vi "OriginSearch.vi"(8 "error in":errorcluster, 11 "VISA resource":refnum<visa-resource-name>) -> (0 "error out":errorcluster)   [LabVIEW 2012, in "Micos_uic.lvlib"]
uses:
  <instrlib>/Micos_uic/Micos_uic.lvlib
  <vilib>/Utility/error.llb/DialogType.ctl
panel:
  out "Itration":i32
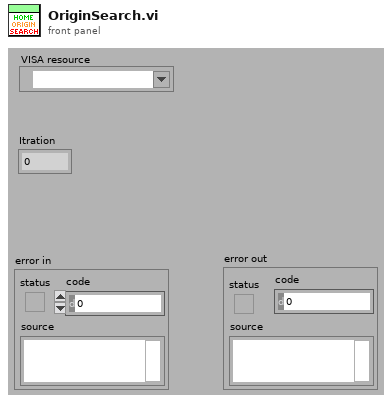
[diagram p1: front panel]
types:
  T1 = typedef "DialogType.ctl" = u16
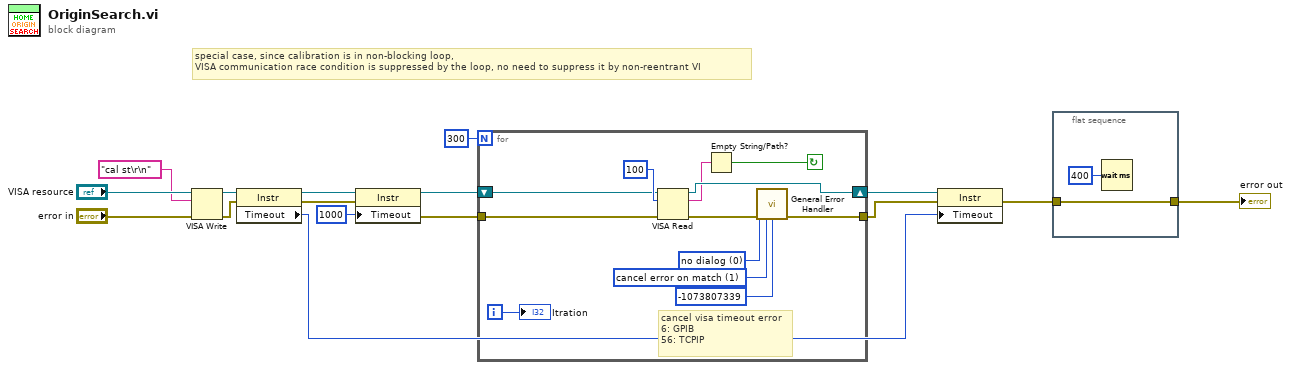
[diagram p0: block diagram]
diagram:
  # "special case, since calibration is in non-blocking loop,\nVISA communication race condition is suppressed by the loop, no need to suppress it by non-reentrant VI"
  n1 = VISA Write(VISA resource name="VISA resource", write buffer="cal st\r\n", error in (no error)="error in") -> (VISA resource name out=w13:refnum<visa-resource-name>, error out=w10:errorcluster)  [unwired: 1 out]
  n2 = property class="Instr"(reference=w13, error in=w10) -> (reference out=w12:refnum<visa-resource-name>, error out=w9:errorcluster, "Timeout"=w6:u32)
  n3 = property class="Instr"(reference=w12, error in=w9, "Timeout"=u32 1000 ("General Settings:Timeout Value")) -> (reference out=w11:refnum<visa-resource-name>, error out=w8:errorcluster)
  n4 = for {
    N: 300 -> [_]
    tunnel: w8 -> [w20]
    tunnel: [w25] -> w4
    shift-right: [w26] -> w7
    shift-left: w11 -> [w19]
    i -> [w18]
    stop <- w21 continue-if-true
    w17 = T1 0 items=["no dialog", "OK message", "continue or stop message", "OK message + warnings", "continue/stop + warnings"] ("type of dialog (OK msg:1)")
    w24 = 1 items=["no exception", "cancel error on match", "set error on match"] ("[exception action] (none:0)")
    # "cancel visa timeout error\n6: GPIB\n56: TCPIP"
    n5 = VISA Read(VISA resource name=w19, byte count=u32 100, error in (no error)=w20) -> (VISA resource name out=w26:refnum<visa-resource-name>, read buffer=w22:string, error out=w28:errorcluster)  [unwired: 1 out]
    n6 = Empty String/Path?(string/path=w22) -> (empty?=w21:bool)
    n7 = call <vilib>:"General Error Handler.vi"("type of dialog (OK msg:1)"=w17, "error in (no error)"=w28, "[exception action] (none:0)"=w24, "[exception code]"=-1073807339) -> ("error out"=w25:errorcluster)  [unwired: 7 in, 4 out]
    "Itration" <- w18
  }
  n8 = property class="Instr"(reference=w7, error in=w4, "Timeout"=w6) -> (error out=w1:errorcluster)  [unwired: 1 out]
  n9 = flat-sequence {
    tunnel: [w29] -> w2
    tunnel: w1 -> [w29]
    frame #0 {
      n10 = Wait (ms)(milliseconds to wait=u32 400) -> ()  [unwired: 1 out]
    }
  }
  "error out" <- w2
